vi "AlliGator Get Python Script Function List.vi"(8 "error in (no error)":errorcluster, 11 "File Path":path) -> (0 "error out":errorcluster, 1 "Parent Menu Locations":string[](array[string]), 3 "Array of Python Functions Info":T1[](array[typedef]))   [LabVIEW 2021, in "AlliGator Python Plugins.lvlib"]
doc: "Extracts list of python plugin functions and their information from python script."
uses:
  AlliGator Python Plugins.lvlib
  AlliGator Python Function Information.ctl
  AlliGator Python Function Parameter Definition.ctl
  AlliGator Python Function Output Definition.ctl
  AlliGator Python Plugin Target Type.ctl
  <userlib>/_OpenG.lib/string/string.llb/openg_string.lvlib
  Strings/Strings.lvlib
  Error/Error.lvlib
panel:
  # "see the AlliGator License on the block diagram (Ctrl+E or Window:Show Block Diagram)"
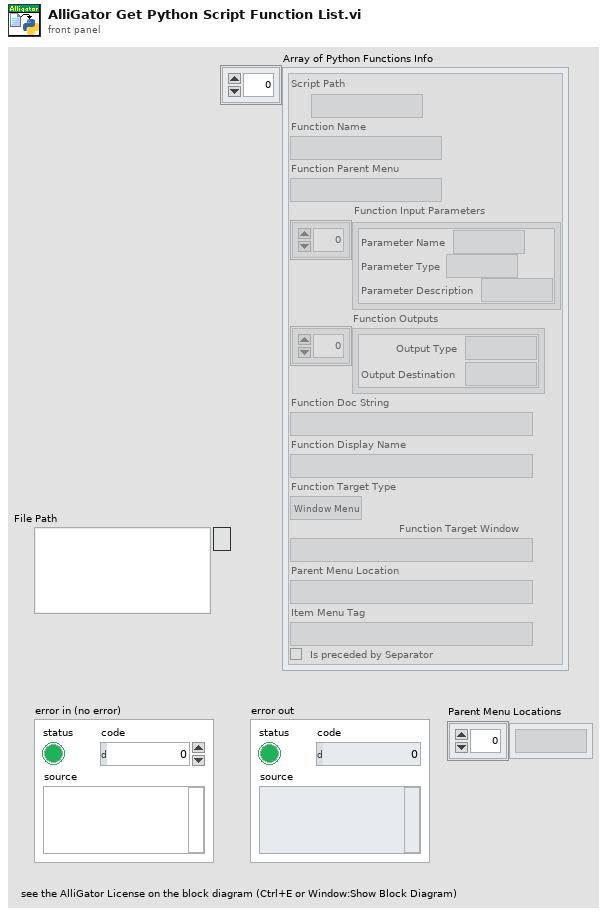
[diagram p1: front panel]
types:
  T1 = typedef "AlliGator Python Plugins.lvlib/AlliGator Python Function Information.ctl" = cluster{"Script Path":path, "Function Name":string, "Function Parent Menu":string, "Function Input Parameters":T2[], "Function Outputs":T3[], "Function Doc String":string, "Function Display Name":string, "Function Target Type":T4, "Function Target Window":string, "Parent Menu Location":string, "Item Menu Tag":string, "Is preceded by Separator":bool}
  T2 = typedef "AlliGator Python Plugins.lvlib/AlliGator Python Function Parameter Definition.ctl" = cluster{"Parameter Name":string, "Parameter Type":string, "Parameter Description":string}
  T3 = typedef "AlliGator Python Plugins.lvlib/AlliGator Python Function Output Definition.ctl" = cluster{"Output Type":string, "Output Destination":string}
  T4 = typedef "AlliGator Python Plugins.lvlib/AlliGator Python Plugin Target Type.ctl" = enum16{"Undefined", "Window Menu", "Object Menu"}
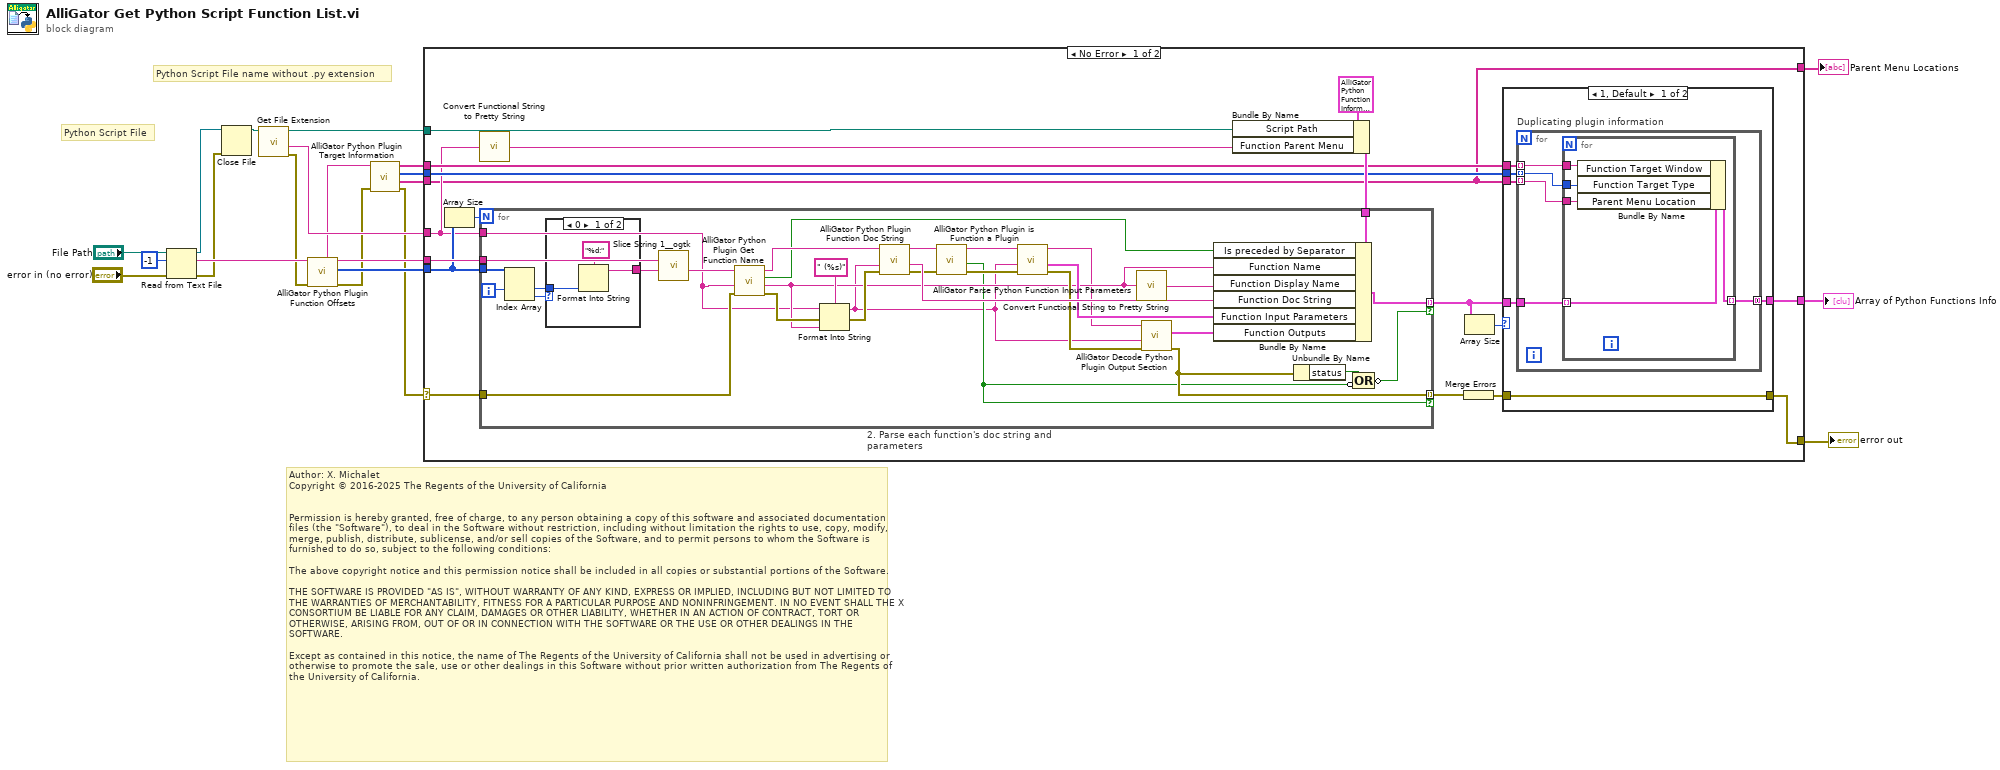
[diagram p0: block diagram]
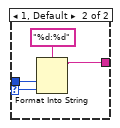
[diagram p3: hidden frame]
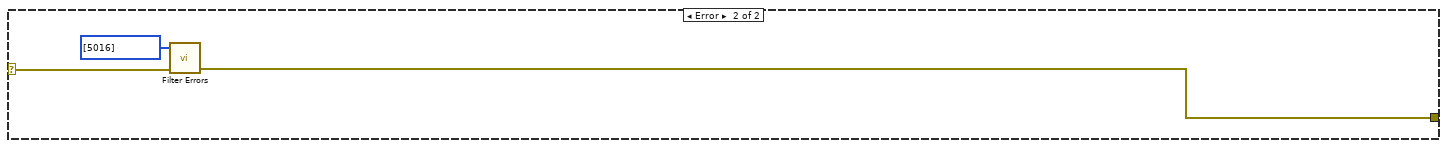
[diagram p4: hidden frame]
diagram:
  # "Author: X. Michalet\nCopyright © 2016-2025 The Regents of the University of California\n \n\nPermission is hereby granted, free of charge, to any person obtaining a copy of this software and associated documentation files (the \"Software\"), to deal in the Software without restriction, including without limitation the rights to use, copy, modify, merge, publish, distribute, sublicense, and/or sell copies of the Software, and to permit persons to whom the Software is furnished to do so, subject to the following conditions:\n\nThe above copyright notice and this permission notice shall be included in all copies or substantial portions of the Software.\n\nTHE SOFTWARE IS PROVIDED \"AS IS\", WITHOUT WARRANTY OF ANY KIND, EXPRESS OR IMPLIED, INCLUDING BUT NOT LIMITED TO THE WARRANTIES OF MERCHANTABILITY, FITNESS FOR A PARTICULAR PURPOSE AND NONINFRINGEMENT. IN NO EVENT SHALL THE X CONSORTIUM BE LIABLE FOR ANY CLAIM, DAMAGES OR OTHER LIABILITY, WHETHER IN AN ACTION OF CONTRACT, TORT OR OTHERWISE, ARISING FROM, OUT OF OR IN CONNECTION WITH THE SOFTWARE OR THE USE OR OTHER DEALINGS IN THE SOFTWARE.\n\nExcept as contained in this notice, the name of The Regents of the University of California shall not be used in advertising or otherwise to promote the sale, use or other dealings in this Software without prior written authorization from The Regents of the University of California."
  # "Python Script File name without .py extension"
  # "Python Script File"
  n1 = Read from Text File(file (use dialog)="File Path", count=-1, error in="error in (no error)") -> (refnum out=w19:refnum<file>, text=w15:string, error out=w12:errorcluster)  [unwired: 1 in, 1 out]
  n2 = Close File(refnum=w19, error in=w12) -> (path=w17:path)  [unwired: 1 out]
  n3 = call <vilib>:"Get File Extension.vi"("file"=w17) -> ("error out"=w11:errorcluster, "filename without extension"=w10:string, "dup file"=w16:path)  [unwired: 6 in, 2 out]
  n4 = call "AlliGator Python Plugin Function Offsets.vi"("Error In"=w11, "String in"=w15) -> ("Error Out"=w8:errorcluster, "Function Offsets"=w13:i32[], "String in (dup)"=w14:string, "Script Header"=w9:string)  [unwired: 6 in]
  n5 = call "AlliGator Python Plugin Target Information.vi"("error in (no error)"=w8, "Script Header"=w9) -> ("error out"=w7:errorcluster, "Parent Menu Locations"=w3:string[], "Function Target Types"=w4:T4[], "Function Target Windows"=w5:string[])  [unwired: 6 in]
  n6 = case shown="No Error" w7 {
    selector: w7 -> [w33 w98]
    tunnel: w16 -> [w37 _]
    tunnel: w14 -> [w36 _]
    tunnel: w13 -> [w35 _]
    tunnel: w10 -> [w26 _]
    tunnel: [w24 w96] -> w6
    tunnel: w5 -> [w31 _]
    tunnel: w4 -> [w30 _]
    tunnel: w3 -> [w22 _]
    tunnel: [w29 _] -> w2
    tunnel: [w22 _] -> w1
    frame No Error {
      n7 = Array Size(array=w35) -> (size(s)=w34:i32)
      n8 = call "Convert Functional String to Pretty String.vi"("Functional Name"=w26) -> ("Pretty Name"=w23:string)  [unwired: 4 in]
      n9 = Bundle By Name(cluster=T1 {"Script Path"=path "", "Function Name"="", "Function Parent Menu"="", "Function Input Parameters"=[], "Function Outputs"=[], "Function Doc String"="", "Function Display Name"="", "Function Target Type"=enum."Window Menu", "Function Target Window"="", "Parent Menu Location"="", "Item Menu Tag"="", "Is preceded by Separator"=FALSE} ("Array of Python Functions Info"), "Script Path"=w37, "Function Parent Menu"=w23) -> (w38:T1)
      n10 = for "2. Parse each function's doc string and parameters" {
        N: w34 -> [_]
        tunnel: w36 -> [w86]
        tunnel: w38 -> [w88]
        tunnel: [w87] -> w28 mode=indexing if=w65
        tunnel: w35 -> [w85]
        tunnel: w26 -> [w57]
        tunnel: w33 -> [w78]
        tunnel: [w67] -> w32 mode=indexing if=w61
        i -> [w84]
        n11 = Index Array(array=w85, index #1=w84) -> (element #1=w83:i32, element #2=w82:i32)  [unwired: 1 in]
        n12 = case shown="0" w82 {
          selector: w82 -> [_ w94]
          tunnel: w83 -> [w91 w95]
          tunnel: [w89 w92] -> w81
          frame 0 {
            n13 = Format Into String(format string="%d:", w91) -> (resulting string=w89:string)  [unwired: 2 in, 1 out]
          }
          frame 1, Default {
            n14 = Format Into String(format string="%d:%d", w95, w94) -> (resulting string=w92:string)  [unwired: 2 in, 1 out]
          }
        }
        n15 = call <userlib>:"Slice String 1__ogtk.vi"("Subset (i:j)"=w81, "String"=w86) -> ("Substring (String[i:j])"=w80:string)  [unwired: 7 in]
        n16 = call "AlliGator Python Plugin Get Function Name.vi"("Error In"=w78, "Source"=w57, "String in"=w80) -> ("Error Out"=w76:errorcluster, "function_name"=w64:string, "Is preceded by Separator"=w60:bool, "String out"=w79:string)  [unwired: 5 in]
        n17 = Format Into String(format string=" (%s)", initial string=w57, error in=w76, w64) -> (resulting string=w58:string, error out=w75:errorcluster)
        n18 = call "AlliGator Python Plugin Function Doc String.vi"("Error In"=w75, "Source"=w58, "String in"=w79) -> ("Error Out"=w72:errorcluster, "Doc String"=w73:string, "String out"=w77:string)  [unwired: 6 in]
        n19 = call "AlliGator Python Plugin is Function a Plugin.vi"("Error In"=w72, "String in"=w77) -> ("Error Out"=w71:errorcluster, "Is AlliGator Python Plugin?"=w61:bool, "String out"=w70:string)  [unwired: 7 in]
        n20 = call "AlliGator Parse Python Function Input Parameters.vi"("Error In"=w71, "Source"=w58, "Input String"=w70) -> ("Error Out"=w69:errorcluster, "Function Input Parameters"=w68:T2[], "Output string"=w59:string)  [unwired: 6 in]
        n21 = call "Convert Functional String to Pretty String.vi"("Functional Name"=w64) -> ("Pretty Name"=w63:string)  [unwired: 4 in]
        n22 = call "AlliGator Decode Python Plugin Output Section.vi"("error in (no error)"=w69, "Source"=w58, "Input String"=w59) -> ("error out"=w67:errorcluster, "Function Outputs"=w62:T3[])  [unwired: 6 in, 1 out]
        n23 = Bundle By Name(cluster=w88, "Is preceded by Separator"=w60, "Function Name"=w64, "Function Display Name"=w63, "Function Doc String"=w73, "Function Input Parameters"=w68, "Function Outputs"=w62) -> (w87:T1)
        n24 = Unbundle By Name(w67) -> ("status"=w66:bool)
        n25 = Compound Arithmetic op=OR(w66, invert w61) -> (invert w65:bool)
      }
      n26 = Merge Errors(w32) -> (w25:errorcluster)
      n27 = Array Size(array=w28) -> (size(s)=w27:i32)
      n28 = case shown="1, Default" w27 {
        tunnel: w31 -> [w43 _]
        tunnel: w30 -> [w45 _]
        tunnel: w22 -> [w44 _]
        tunnel: w28 -> [w42 w56]
        tunnel: [w41 w56] -> w29
        tunnel: w25 -> [w40 _]
        tunnel: [w40 _] -> w24
        frame 1, Default {
          n29 = for "Duplicating plugin information" {
            tunnel: w45 -> [w48] mode=indexing
            tunnel: w44 -> [w47] mode=indexing
            tunnel: w43 -> [w49] mode=indexing
            tunnel: w42 -> [w50]
            tunnel: [w46] -> w41 mode=concatenating
            n30 = for {
              tunnel: w50 -> [w55] mode=indexing
              tunnel: w49 -> [w54]
              tunnel: w48 -> [w53]
              tunnel: w47 -> [w52]
              tunnel: [w51] -> w46 mode=indexing
              n31 = Bundle By Name(cluster=w55, "Function Target Window"=w54, "Function Target Type"=w53, "Parent Menu Location"=w52) -> (w51:T1)
            }
          }
        }
        frame 0 {
        }
      }
    }
    frame Error {
      n32 = call "Filter Errors.vi"("Filtered Errors"=i32[] [5016], "error in (no error)"=w98) -> ("error out"=w96:errorcluster)  [unwired: 7 in]
    }
  }
  "error out" <- w6
  "Array of Python Functions Info" <- w2
  "Parent Menu Locations" <- w1
